vi "Get Card Name.vi"(8 "error in (no error)":errorcluster, 10 "Slot #":i32=1, 11 "Slot 1 Module Type":T1) -> (0 "error out":errorcluster, 3 "resulting string":string)   [LabVIEW 2017]
uses:
  Module Type.ctl
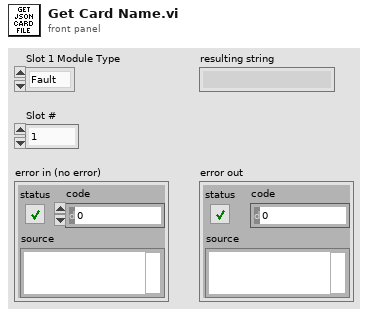
[diagram p1: front panel]
types:
  T1 = typedef "Module Type.ctl" = enum16{"Fault", "Instrument"}
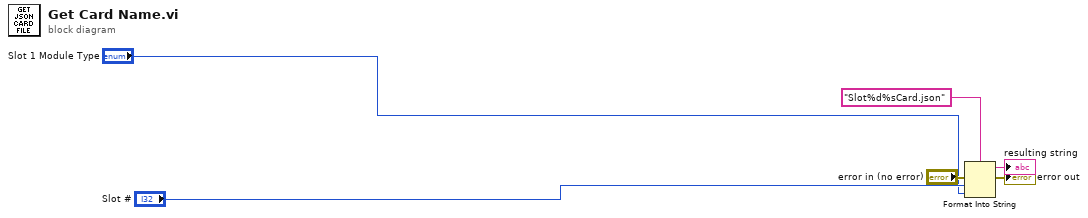
[diagram p0: block diagram]
diagram:
  n1 = Format Into String(format string="Slot%d%sCard.json", error in="error in (no error)", "Slot #", "Slot 1 Module Type") -> (resulting string=→"resulting string":string, error out=→"error out":errorcluster)  [unwired: 1 in]
